vi "getElementType.vi"(8 "error in (no error)":errorcluster, 10 "Name":string, 11 "tBSONDocument in":refnum<class "tBSONDocument.lvclass">) -> (0 "error out":errorcluster, 2 "TypeClass":string, 3 "tBSONDocument out":refnum<class "tBSONDocument.lvclass">)   [LabVIEW 2013, in "BSON.lvlib" / "tBSONDocument.lvclass"]
doc: "Returns the class name of the element with a given name. Can be used to determine the structure of a document."
uses:
  tBSONDocument.lvclass
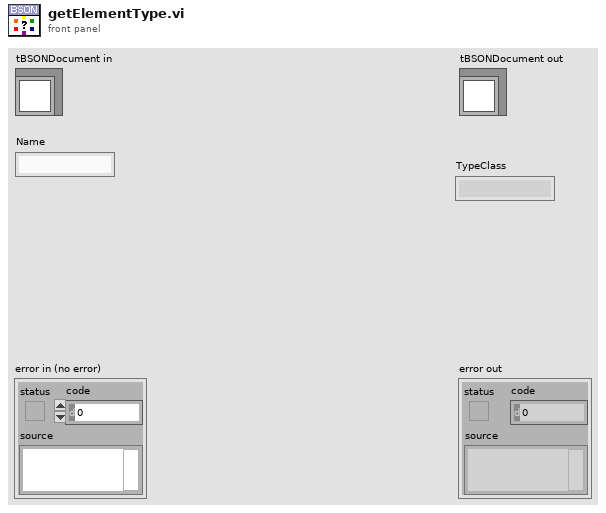
[diagram p1: front panel]
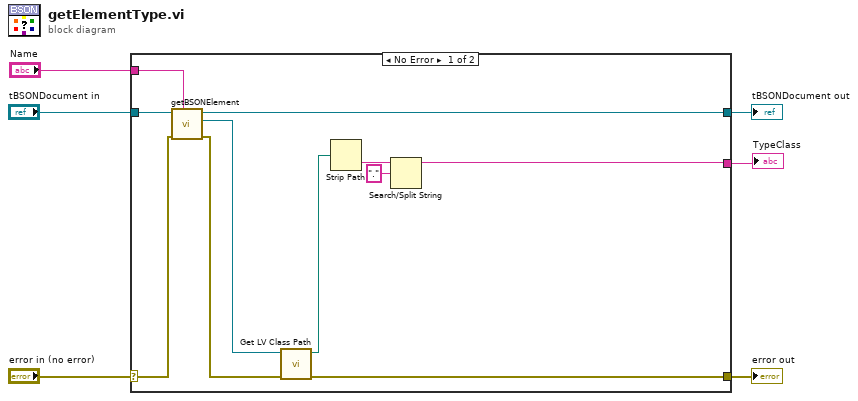
[diagram p0: block diagram]
diagram:
  n1 = case shown="No Error" "error in (no error)" {
    selector: "error in (no error)" -> [w16 w19]
    tunnel: [w12 w19] -> w5
    tunnel: [w15 w18] -> w3
    tunnel: "tBSONDocument in" -> [w17 w18]
    tunnel: "Name" -> [w7 _]
    tunnel: [w8 _] -> w1
    frame No Error {
      n2 = call "getBSONElement.vi"("Name"=w7, "error in (no error)"=w16, "tBSONDocument in"=w17) -> ("error out"=w13:errorcluster, "Element"=w14:refnum<class "tBSONElement.lvclass">, "tBSONDocument out"=w15:refnum<class "tBSONDocument.lvclass">)  [unwired: 6 in]
      n3 = call <vilib>:"Get LV Class Path.vi"("error in (no error)"=w13, "object"=w14) -> ("error out"=w12:errorcluster, "class path"=w11:path)  [unwired: 8 in]
      n4 = Strip Path(path=w11) -> (name=w10:string)  [unwired: 1 out]
      n5 = Search/Split String(string=w10, search string/char (-)=".") -> (substring before match=w8:string)  [unwired: 1 in, 2 out]
    }
    frame Error {
    }
  }
  "error out" <- w5
  "tBSONDocument out" <- w3
  "TypeClass" <- w1
